vi "Target.vi"   [LabVIEW 2025]
uses:
  <vilib>/eio/utilities/niEioResolveVilibRelativePath.vi
  <vilib>/rvi/interface/RandomDataEmulation/niFpgaRandomDataHandleErrors.vi
  <vilib>/rvi/Memory/Memory_Emulation/nirvimemoryFastEmulation.vi
  <vilib>/rvi/Memory/Memory_Emulation/nirvimemoryEmulation.vi
  <vilib>/rvi/Emulation/niFpgaEmulationIsFPGAContextNoSignature.vi
  <vilib>/rvi/DataTransferAndStorage/Container/Common/niFpgaContainerGetUniqueNameForEmu.vi
  <vilib>/rvi/Emulation/niFpgaProcessEmulError.vi
  <vilib>/rvi/Emulation/niFpgaSctlEmulationGetInTimedLoop.vi
  <vilib>/rvi/errors/nirviReportUnexpectedCaseInternalError (U32).vi
  <vilib>/ARTS-Lab/Array-based Linear Algebra/matrix_matrix_VIs/matrix_matrix_multiply_SGL.vi
  <vilib>/rvi/DataTransferAndStorage/Container/XNode/niFpgaContainer.xnode
  <vilib>/rvi/interface/RandomDataEmulation/nirviRandomDataFpgaReadWriteTemplate.vi
  <vilib>/ARTS-Lab/Array-based Linear Algebra/vector_matrix_multiply_VIs/vector_matrix_multiply_SGL.vi
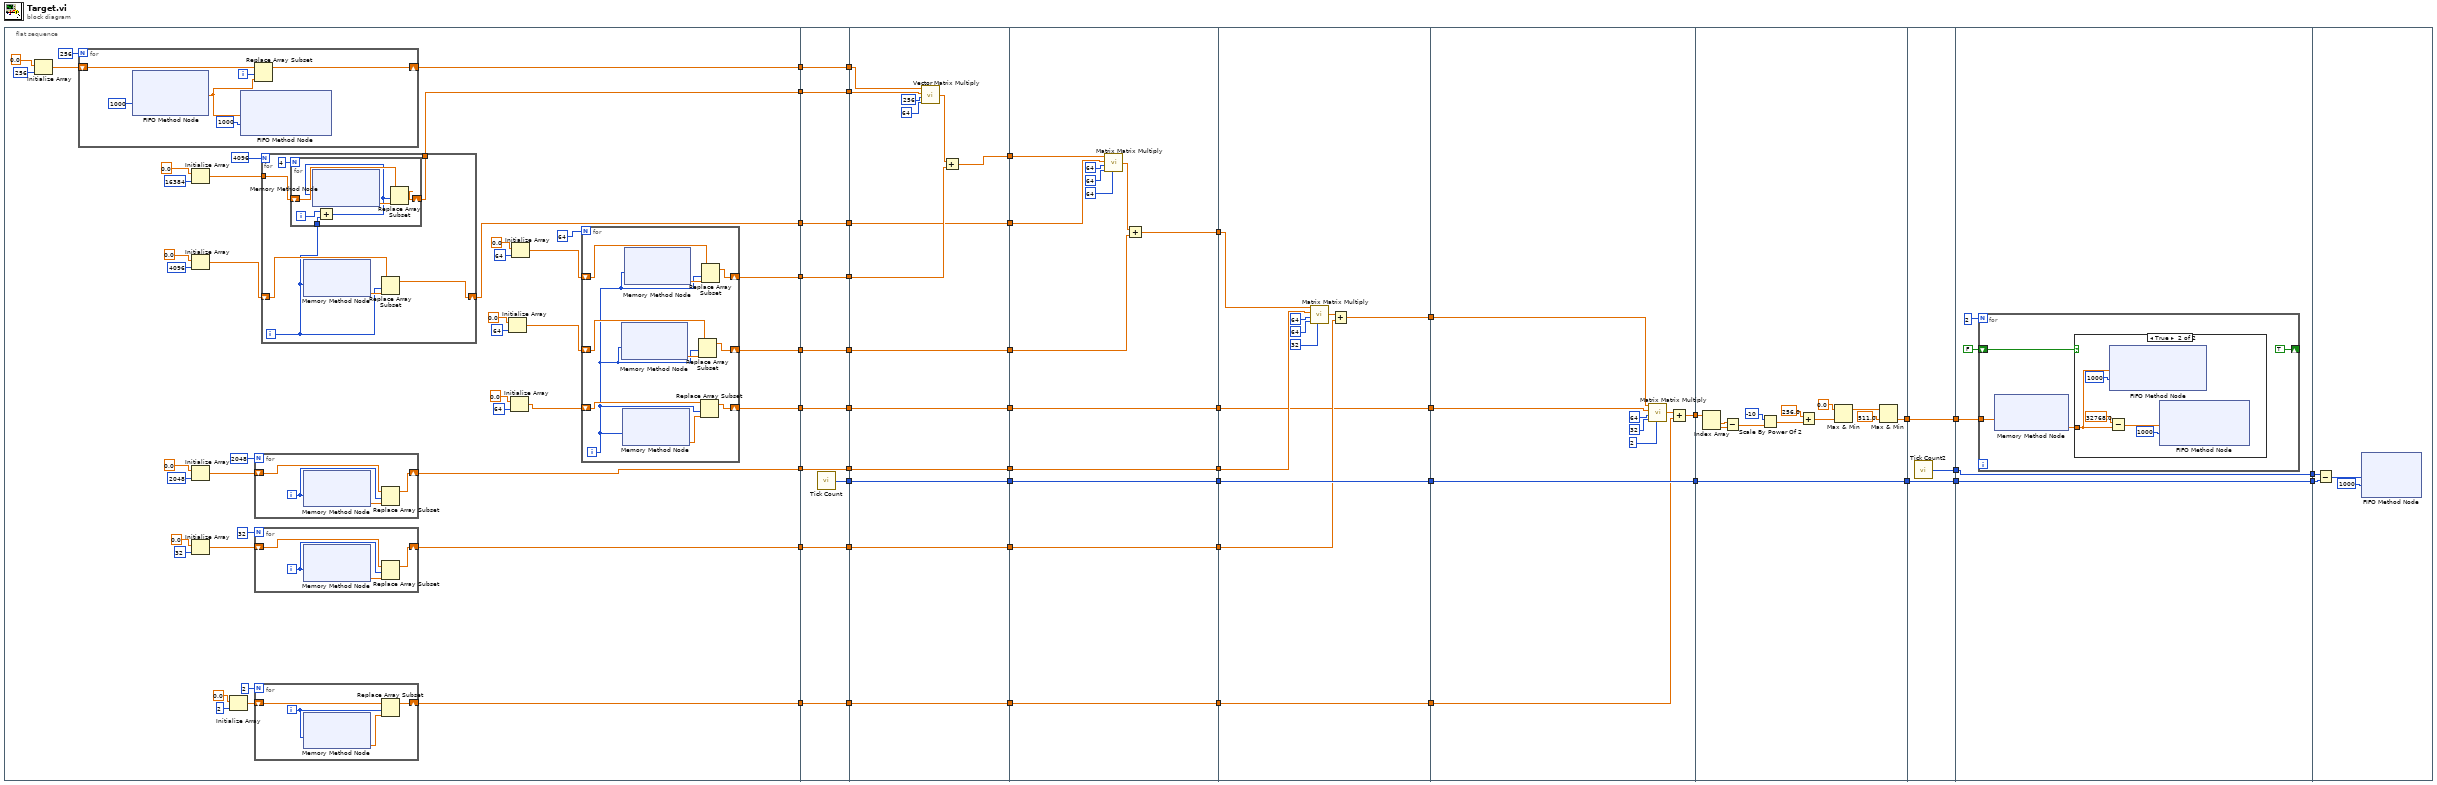
[diagram p0: block diagram]
diagram:
  n1 = flat-sequence {
    tunnel: [w87] -> w37
    tunnel: [w57] -> w33
    tunnel: [w56] -> w24
    tunnel: [w52] -> w22
    tunnel: [w51] -> w21
    tunnel: [w50] -> w18
    tunnel: [w49] -> w14
    tunnel: [w48] -> w10
    tunnel: [w47] -> w5
    tunnel: w37 -> [w139]
    tunnel: [w139] -> w35
    tunnel: [w138] -> w36
    tunnel: [w137] -> w34
    tunnel: w33 -> [w137]
    tunnel: [w136] -> w25
    tunnel: w24 -> [w136]
    tunnel: [w135] -> w23
    tunnel: w22 -> [w135]
    tunnel: w21 -> [w134]
    tunnel: [w134] -> w20
    tunnel: w18 -> [w133]
    tunnel: [w133] -> w17
    tunnel: w14 -> [w132]
    tunnel: [w132] -> w13
    tunnel: w10 -> [w131]
    tunnel: [w131] -> w9
    tunnel: w5 -> [w130]
    tunnel: [w130] -> w4
    tunnel: w36 -> [w153]
    tunnel: [w153] -> w32
    tunnel: w35 -> [w148]
    tunnel: [w149] -> w31
    tunnel: w34 -> [w147]
    tunnel: [w146] -> w26
    tunnel: w25 -> [w146]
    tunnel: w23 -> [w145]
    tunnel: w20 -> [w144]
    tunnel: [w144] -> w19
    tunnel: w17 -> [w143]
    tunnel: [w143] -> w16
    tunnel: w13 -> [w142]
    tunnel: [w142] -> w12
    tunnel: w9 -> [w141]
    tunnel: [w141] -> w8
    tunnel: w4 -> [w140]
    tunnel: [w140] -> w3
    tunnel: w32 -> [w166]
    tunnel: [w166] -> w30
    tunnel: w31 -> [w160]
    tunnel: [w161] -> w28
    tunnel: w26 -> [w159]
    tunnel: w19 -> [w158]
    tunnel: w16 -> [w157]
    tunnel: [w157] -> w15
    tunnel: w12 -> [w156]
    tunnel: [w156] -> w11
    tunnel: w8 -> [w155]
    tunnel: [w155] -> w7
    tunnel: w3 -> [w154]
    tunnel: [w154] -> w2
    tunnel: w30 -> [w177]
    tunnel: [w177] -> w29
    tunnel: w28 -> [w171]
    tunnel: [w172] -> w27
    tunnel: w15 -> [w170]
    tunnel: w11 -> [w169]
    tunnel: w7 -> [w168]
    tunnel: [w168] -> w6
    tunnel: w2 -> [w167]
    tunnel: [w167] -> w1
    tunnel: [w181] -> w46
    tunnel: [w186] -> w45
    tunnel: w29 -> [w186]
    tunnel: w27 -> [w180]
    tunnel: w6 -> [w179]
    tunnel: w1 -> [w178]
    tunnel: w46 -> [w189]
    tunnel: [w188] -> w44
    tunnel: w45 -> [w187]
    tunnel: [w187] -> w43
    tunnel: w44 -> [w202]
    tunnel: [w202] -> w42
    tunnel: w43 -> [w201]
    tunnel: [w201] -> w41
    tunnel: [w200] -> w40
    tunnel: w42 -> [w206]
    tunnel: [w203] -> w39
    tunnel: w41 -> [w204]
    tunnel: [w204] -> w38
    tunnel: w40 -> [w203]
    tunnel: w39 -> [w220]
    tunnel: w38 -> [w219]
    frame #0 {
      n2 = Initialize Array(sgl 0.0 ("element"), 256 ("dimension size")) -> (w84:sgl[])
      n3 = for {
        N: 256 -> [_]
        shift-right: [w125] -> w87
        shift-left: w84 -> [w127]
        i -> [w124]
        n4 = xnode ("FIFO Method Node")("Timeout"=1000) -> ("Element"=w126:sgl)  [unwired: 1 in, 2 out]
        n5 = xnode ("FIFO Method Node")("Element"=w126, "Timeout"=1000) -> ()  [unwired: 1 in, 2 out]
        n6 = Replace Array Subset(array=w127, new element=w126, index=w124) -> (w125:sgl[])
      }
      n7 = Initialize Array(sgl 0.0 ("element"), 16384 ("dimension size")) -> (w53:sgl[])
      n8 = Initialize Array(sgl 0.0 ("element"), 4096 ("dimension size")) -> (w54:sgl[])
      n9 = Initialize Array(sgl 0.0 ("element"), 2048 ("dimension size")) -> (w64:sgl[])
      n10 = Initialize Array(sgl 0.0 ("element"), 32 ("dimension size")) -> (w62:sgl[])
      n11 = Initialize Array(sgl 0.0 ("element"), 2 ("dimension size")) -> (w63:sgl[])
      n12 = for {
        N: 2048 -> [_]
        shift-right: [w122] -> w50
        shift-left: w64 -> [w121]
        i -> [w120]
        n13 = xnode ("Memory Method Node")("Address"=w120) -> ("Data"=w123:sgl)  [unwired: 1 in, 1 out]
        n14 = Replace Array Subset(array=w121, new element=w123, index=w120) -> (w122:sgl[])
      }
      n15 = for {
        N: 32 -> [_]
        shift-right: [w117] -> w49
        shift-left: w62 -> [w118]
        i -> [w116]
        n16 = xnode ("Memory Method Node")("Address"=w116) -> ("Data"=w119:sgl)  [unwired: 1 in, 1 out]
        n17 = Replace Array Subset(array=w118, new element=w119, index=w116) -> (w117:sgl[])
      }
      n18 = for {
        N: 2 -> [_]
        shift-right: [w113] -> w47
        shift-left: w63 -> [w114]
        i -> [w112]
        n19 = xnode ("Memory Method Node")("Address"=w112) -> ("Data"=w115:sgl)  [unwired: 1 in, 1 out]
        n20 = Replace Array Subset(array=w114, new element=w115, index=w112) -> (w113:sgl[])
      }
      n21 = for {
        N: 4096 -> [_]
        shift-right: [w93] -> w51
        shift-left: w54 -> [w91]
        tunnel: w53 -> [w92]
        tunnel: [w89] -> w52
        i -> [w90]
        n22 = for {
          N: 4 -> [_]
          shift-right: [w100] -> w89
          shift-left: w92 -> [w99]
          tunnel: w90 -> [w97]
          i -> [w98]
          n23 = Add(x=w98, y=w97) -> (x+y=w96:i32)
          n24 = xnode ("Memory Method Node")("Address"=w96) -> ("Data"=w101:sgl)  [unwired: 1 in, 1 out]
          n25 = Replace Array Subset(array=w99, new element=w101, index=w96) -> (w100:sgl[])
        }
        n26 = xnode ("Memory Method Node")("Address"=w90) -> ("Data"=w95:sgl)  [unwired: 1 in, 1 out]
        n27 = Replace Array Subset(array=w91, new element=w95, index=w90) -> (w93:sgl[])
      }
      n28 = Initialize Array(sgl 0.0 ("element"), 64 ("dimension size")) -> (w59:sgl[])
      n29 = Initialize Array(sgl 0.0 ("element"), 64 ("dimension size")) -> (w58:sgl[])
      n30 = Initialize Array(sgl 0.0 ("element"), 64 ("dimension size")) -> (w60:sgl[])
      n31 = for {
        N: 64 -> [_]
        shift-right: [w107] -> w57
        shift-left: w60 -> [w108]
        shift-right: [w103] -> w56
        shift-left: w59 -> [w106]
        shift-right: [w104] -> w48
        shift-left: w58 -> [w105]
        i -> [w102]
        n32 = xnode ("Memory Method Node")("Address"=w102) -> ("Data"=w110:sgl)  [unwired: 1 in, 1 out]
        n33 = xnode ("Memory Method Node")("Address"=w102) -> ("Data"=w109:sgl)  [unwired: 1 in, 1 out]
        n34 = xnode ("Memory Method Node")("Address"=w102) -> ("Data"=w111:sgl)  [unwired: 1 in, 1 out]
        n35 = Replace Array Subset(array=w106, new element=w110, index=w102) -> (w103:sgl[])
        n36 = Replace Array Subset(array=w105, new element=w109, index=w102) -> (w104:sgl[])
        n37 = Replace Array Subset(array=w108, new element=w111, index=w102) -> (w107:sgl[])
      }
    }
    frame #1 {
      n38 = call "Tick Count"() -> ("Tick Count(uSec)"=w138:u32)
    }
    frame #2 {
      n39 = call-poly <vilib>:"Vector Matrix Multiply.vi"("p"=64, "n"=256, "B"=w145, "A"=w148) -> ("C"=w152:sgl[])
      n40 = Add(x=w152, y=w147) -> (x+y=w149:sgl[])
    }
    frame #3 {
      n41 = call-poly <vilib>:"Matrix Matrix Multiply.vi"("p"=64 ("n"), "n"=64, "m"=64, "B"=w158, "A"=w160) -> ("C"=w165:sgl[])  [unwired: 1 in]
      n42 = Add(x=w165, y=w159) -> (x+y=w161:sgl[])
    }
    frame #4 {
      n43 = call-poly <vilib>:"Matrix Matrix Multiply.vi"("p"=32, "n"=64, "m"=64, "B"=w170, "A"=w171) -> ("C"=w176:sgl[])  [unwired: 1 in]
      n44 = Add(x=w176, y=w169) -> (x+y=w172:sgl[])
    }
    frame #5 {
      n45 = call-poly <vilib>:"Matrix Matrix Multiply.vi"("p"=2, "n"=32, "m"=64, "B"=w179, "A"=w180) -> ("C"=w183:sgl[])  [unwired: 1 in]
      n46 = Add(x=w183, y=w178) -> (x+y=w181:sgl[])
    }
    frame #6 {
      n47 = Index Array(array=w189) -> (element #1=w194:sgl, element #2=w195:sgl)  [unwired: 2 in]
      n48 = Subtract(x=w194, y=w195) -> (x-y=w196:sgl)
      n49 = Scale By Power Of 2(n=i16 -10, x=w196) -> (x*2^n=w197:sgl)
      n50 = Add(x=sgl 256.0, y=w197) -> (x+y=w198:sgl)
      n51 = Max & Min(x=sgl 0.0, y=w198) -> (max(x,y)=w199:sgl)  [unwired: 1 out]
      n52 = Max & Min(x=w199, y=sgl 511.0) -> (min(x,y)=w188:sgl)  [unwired: 1 out]
    }
    frame #7 {
      n53 = call "Tick Count2"() -> ("Tick Count(uSec)"=w200:u32)
    }
    frame #8 {
      n54 = for {
        N: 2 -> [_]
        tunnel: w206 -> [w211]
        shift-right: [TRUE] -> _
        shift-left: FALSE -> [w210]
        n55 = xnode ("Memory Method Node")("Address"=w211) -> ("Data"=w208:sgl)  [unwired: 1 in, 1 out]
        n56 = case shown="True" w210 {
          tunnel: w208 -> [_ w212]
          frame False {
          }
          frame True {
            n57 = xnode ("FIFO Method Node")("Element"=w212, "Timeout"=1000) -> ()  [unwired: 1 in, 2 out]
            n58 = Subtract(x=sgl 32768.0, y=w212) -> (x-y=w216:sgl)
            n59 = xnode ("FIFO Method Node")("Element"=w216, "Timeout"=1000) -> ()  [unwired: 1 in, 2 out]
          }
        }
      }
    }
    frame #9 {
      n60 = Subtract(x=w220, y=w219) -> (x-y=w218:u32)
      n61 = xnode ("FIFO Method Node")("Element"=w218, "Timeout"=1000) -> ()  [unwired: 1 in, 2 out]
    }
  }
